vi "Teardown.vi"(11 "Teardown in":refnum<class "Teardown.lvclass">) -> (3 "Teardown out":refnum<class "Teardown.lvclass">)   [LabVIEW 2021, in "jettl.lvlib" / "Teardown.lvlib" / "Teardown.lvclass"]
uses:
  Teardown.lvclass
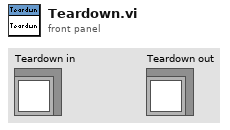
[diagram p1: front panel]
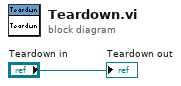
[diagram p0: block diagram]
diagram:
  "Teardown out" <- "Teardown in"
